vi "Timestamp to RFC5322 DateString.vi"(11 "Timestamp (now)":timestamp) -> (3 "RFC5322 Date String":string)   [LabVIEW 2013]
uses:
  RFC5322 Months -- enum.ctl
  <vilib>/regexp/Match Regular Expression.xnode
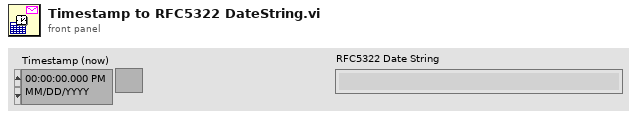
[diagram p1: front panel]
types:
  T1 = typedef "RFC5322 Months -- enum.ctl" = enum16{"Jan", "Feb", "Mar", "Apr", "May", "Jun", "Jul", "Aug", "Sep", "Oct", "Nov", "Dec"}
  T2 = typedef "LVDateTimeRec.ctl" = cluster{"fractional second":dbl, "second":i32, "minute":i32, "hour":i32, "day of month":i32, "month":i32, "year":i32, "day of week":i32, "day of year":i32, "DST":i32}
  T3 = typedef "UTC Offsets -- enum.ctl" = enum16{"UTC-12:00", "UTC-11:00", "UTC-10:00", "UTC-09:30", "UTC-09:00", "UTC-08:00", "UTC-07:00", "UTC-06:00", "UTC-05:00", "UTC-04:00", "UTC-03:30", "UTC-03:00", "UTC-02:00", "UTC-01:00", "UTC-00:00", "UTC+00:00", "UTC+01:00", "UTC+02:00", "UTC+03:00", "UTC+03:30", "UTC+04:00", "UTC+04:30", "UTC+05:00", "UTC+05:30", "UTC+05:45", "UTC+06:00", "UTC+06:30", "UTC+07:00", "UTC+08:00", "UTC+08:45", "UTC+09:00", "UTC+09:30", "UTC+10:00", "UTC+10:30", "UTC+11:00", "UTC+12:00", "UTC+12:45", "UTC+13:00", "UTC+14:00"}
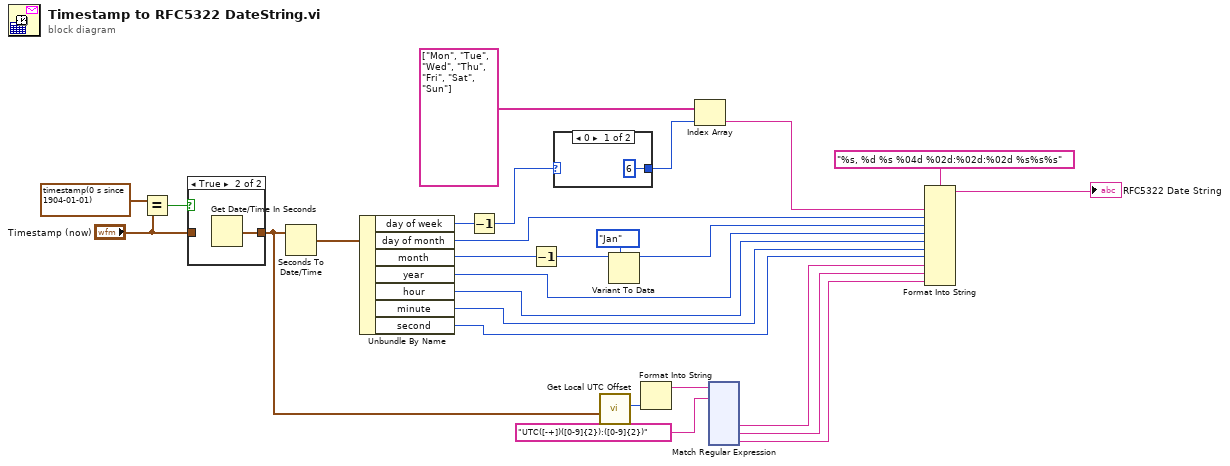
[diagram p0: block diagram]
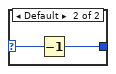
[diagram p2: hidden frame]
diagram:
  n1 = Equal?(x=timestamp(0 s since 1904-01-01), y="Timestamp (now)") -> (x = y?=w19:bool)
  n2 = case shown="True" w19 {
    tunnel: [w28 w29] -> w1
    tunnel: "Timestamp (now)" -> [w28 _]
    frame False {
    }
    frame True {
      n3 = Get Date/Time In Seconds() -> (seconds since 1Jan1904=w29:timestamp)
    }
  }
  n4 = Seconds To Date/Time(time stamp (now)=w1) -> (date time rec=w27:T2)  [unwired: 1 in]
  n5 = Unbundle By Name(w27) -> ("day of week"=w16:i32, "day of month"=w7:i32, "month"=w24:i32, "year"=w5:i32, "hour"=w4:i32, "minute"=w3:i32, "second"=w2:i32)
  n6 = Decrement(x=w16) -> (x-1=w14:i32)
  n7 = Decrement(x=w24) -> (x-1=w21:i32)
  n8 = case shown="0" w14 {
    selector: w14 -> [_ w32]
    tunnel: [6 w31] -> w15
    frame 0 {
    }
    frame Default {
      n9 = Decrement(x=w32) -> (x-1=w31:i32)
    }
  }
  n10 = call "Get Local UTC Offset.vi"("timestamp (now)"=w1) -> ("UTC Offset"=w26:T3)  [unwired: 9 in, 1 out]
  n11 = Variant To Data(type=RFC5322_Months_--_enum."Jan", Variant=w21) -> (data=w6:T1)  [unwired: 1 in, 1 out]
  n12 = Format Into String(w26) -> (resulting string=w25:string)  [unwired: 3 in, 1 out]
  n13 = Index Array(array=string[] ["Mon", "Tue", "Wed", "Thu", "Fri", "Sat", "Sun"], index=w15) -> (element=w13:string)
  n14 = xnode "Match Regular Expression"("input string"=w25, "regular expression"="UTC([-+])([0-9]{2}):([0-9]{2})") -> ("submatch 1"=w10:string, "submatch 2"=w9:string, "submatch 3"=w8:string)  [unwired: 4 in, 5 out]
  n15 = Format Into String(format string="%s, %d %s %04d %02d:%02d:%02d %s%s%s", w13, w7, w6, w5, w4, w3, w2, w10, w9, w8) -> (resulting string=→"RFC5322 Date String":string)  [unwired: 2 in, 1 out]
